vi "REPORT_GEAR_prepare_operations_and_batches_for_csv.vi"(11 "REPORT_GEAR_all_info":T1) -> (2 "report_batches":string[][](array[string]), 3 "report_results":string[][](array[string]))   [LabVIEW 2019]
uses:
  typedef/REPORT_GEAR_all_info.ctl
  typedef/REPORT_GEAR_header_data_display.ctl
  typedef/REPORT_GEAR_statuses.ctl
  _misc/AULocalize/SubVIs/Get Localized Phrase Compact Interface 1D.vi
panel:
  # "GEAR INFO SUMMARY"
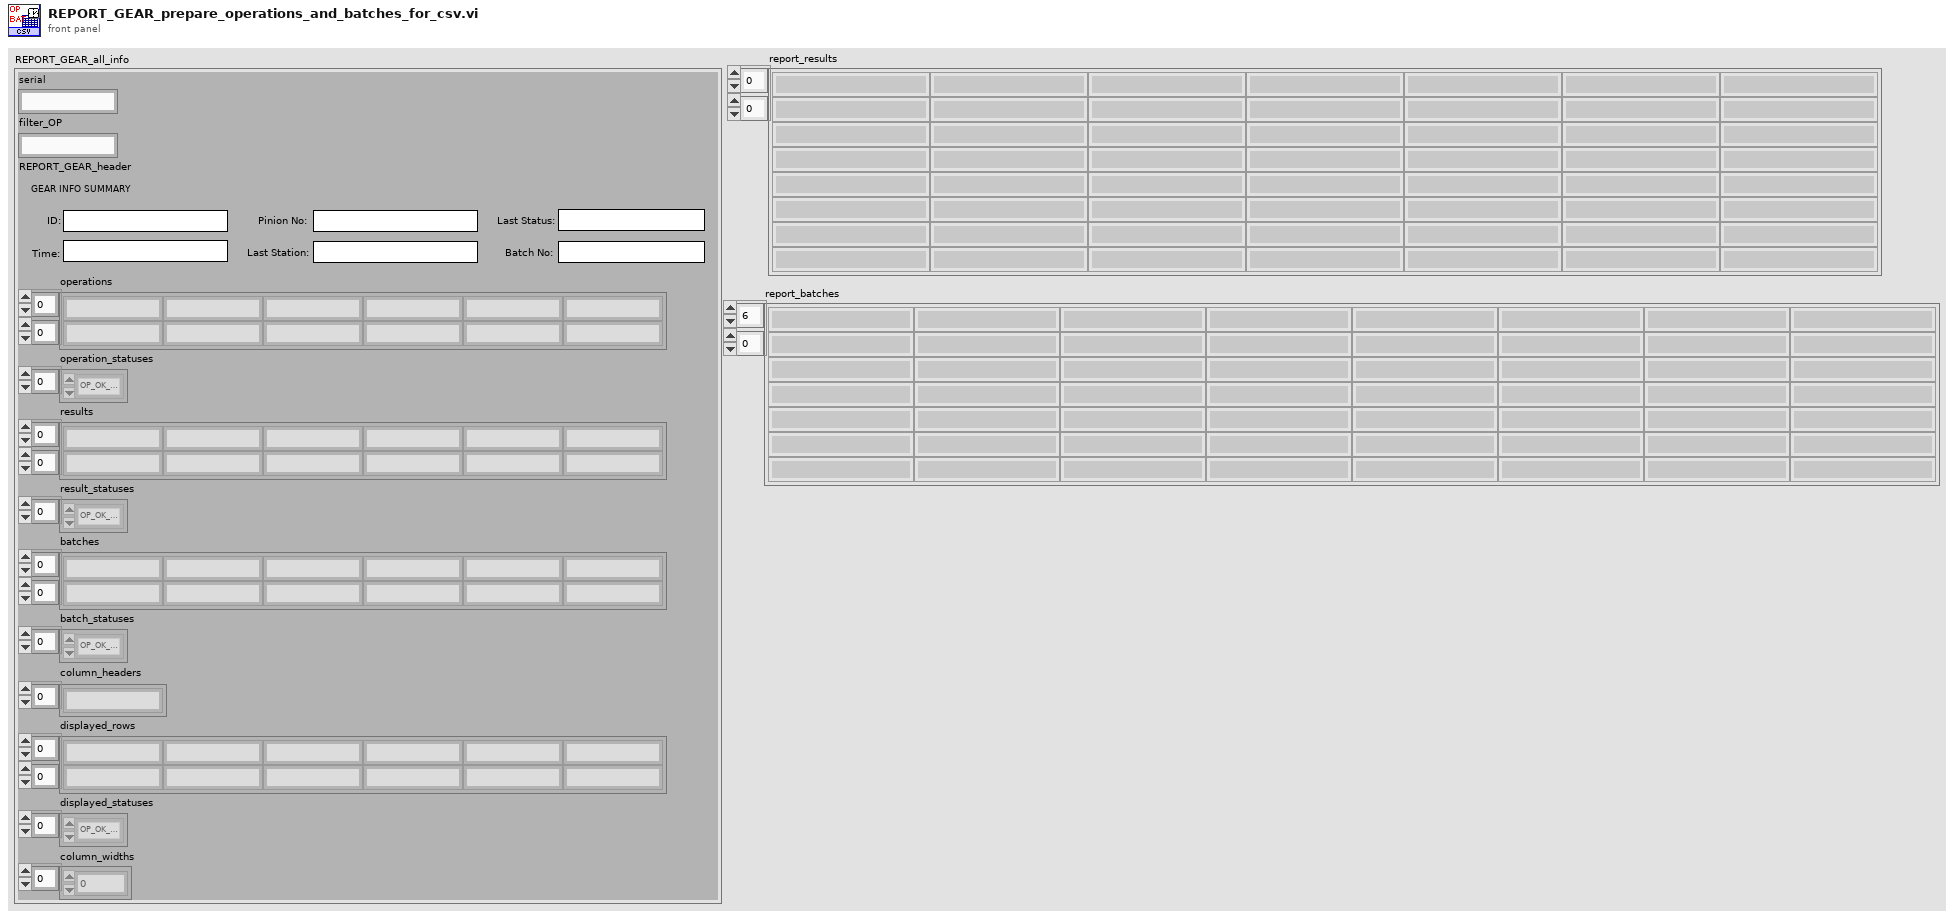
[diagram p1: front panel]
types:
  T1 = typedef "REPORT_GEAR_all_info.ctl" = cluster{"serial":string, "filter_OP":string, "REPORT_GEAR_header":T2, "operations":string[][], "operation_statuses":T3[], "results":string[][], "result_statuses":T3[], "batches":string[][], "batch_statuses":T3[], "column_headers":string[], "displayed_rows":string[][], "displayed_statuses":T3[], "column_widths":i16[]}
  T2 = typedef "REPORT_GEAR_header_data_display.ctl" = cluster{"ID":string, "creation_time":string, "last_station":string, "last_status":string, "pinion_serial":string, "batch_code":string}
  T3 = typedef "REPORT_GEAR_statuses.ctl" = enum16{"OP_OK_hide", "OP_OK_show", "OP_NOK_hide", "OP_NOK_show", "OP_interrupted_hide", "OP_interrupted_show", "OP_in_operation_hide", "OP_in_operation_show", "OP_unexpected_hide", "OP_unexpected_show", "RE_REAL_OK", "RE_REAL_NOK", "RE_STRING", "RE_sub_header", "RE_no_data", "RE_unexpected", "BA_sub_header", "BA_data", "BA_no_data"}
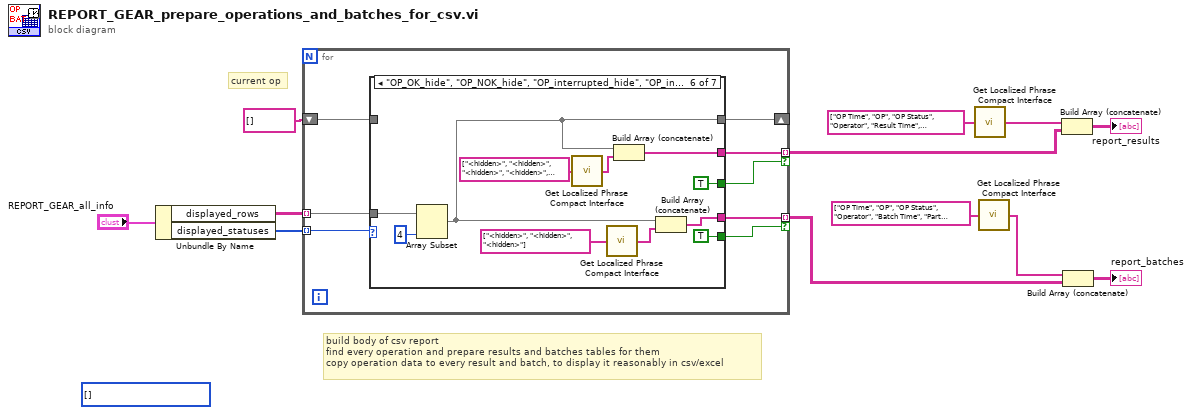
[diagram p0: block diagram]
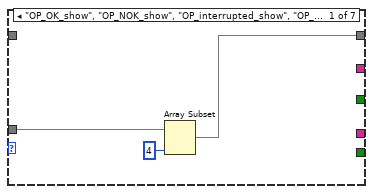
[diagram p2: hidden frame]
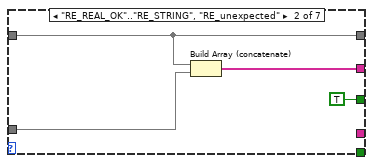
[diagram p3: hidden frame]
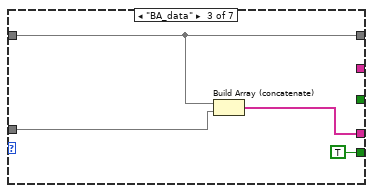
[diagram p4: hidden frame]
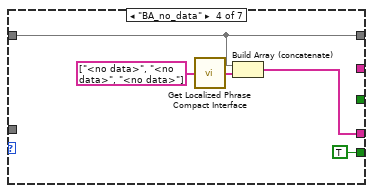
[diagram p5: hidden frame]
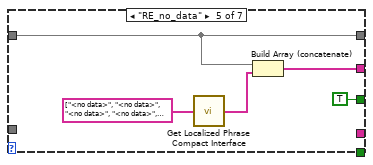
[diagram p6: hidden frame]
diagram:
  (unwired) T3[] [] items=["OP_OK_hide", "OP_OK_show", "OP_NOK_hide", "OP_NOK_show", "OP_interrupted_hide", "OP_interrupted_show", "OP_in_operation_hide", "OP_in_operation_show", "OP_unexpected_hide", "OP_unexpected_show", "RE_REAL_OK", "RE_REAL_NOK", "RE_STRING", "RE_sub_header", "RE_no_data", "RE_unexpected", "BA_sub_header", "BA_data", "BA_no_data"] ("displayed_statuses")
  # "build body of csv report\nfind every operation and prepare results and batches tables for them\ncopy operation data to every result and batch, to display it reasonably in csv/excel"
  # "current op"
  n1 = Unbundle By Name("REPORT_GEAR_all_info") -> ("displayed_rows"=w11:string[][], "displayed_statuses"=w10:T3[])
  n2 = for {
    tunnel: w11 -> [w19] mode=indexing
    tunnel: w10 -> [w20] mode=indexing
    shift-right: [w18] -> _
    shift-left: string[] [] ("displayed_rows") -> [w17]
    tunnel: [w16] -> w4 mode=indexing if=w15
    tunnel: [w14] -> w3 mode=indexing if=w13
    n3 = case shown="\"OP_OK_hide\", \"OP_NOK_hide\", \"OP_interrupted_hide\", \"OP_in_operation_hide\", \"OP_unexpected_hide\"" w20 {
      tunnel: w19 -> [w23 w27 w29 _ _ w43 _]
      tunnel: [w21 w26 w30 w35 w40 w42 w53] -> w18
      tunnel: w17 -> [_ w26 w30 w35 w40 _ w53]
      tunnel: [_ w25 _ _ w38 w51 _] -> w16
      tunnel: [_ TRUE _ _ TRUE TRUE _] -> w15
      tunnel: [_ _ w28 w34 _ w47 _] -> w14
      tunnel: [_ _ TRUE TRUE _ TRUE _] -> w13
      frame "OP_OK_show", "OP_NOK_show", "OP_interrupted_show", "OP_in_operation_show", "OP_unexpected_show" {
        n4 = Array Subset(array=w23, length=4) -> (w21:string[])  [unwired: 1 in]
      }
      frame "RE_REAL_OK".."RE_STRING", "RE_unexpected" {
        n5 = Build Array (concatenate)(w26, w27) -> (w25:string[])
      }
      frame "BA_data" {
        n6 = Build Array (concatenate)(w30, w29) -> (w28:string[])
      }
      frame "BA_no_data" {
        n7 = call-poly "Get Localized Phrase Compact Interface.vi"("Key"=string[] ["<no data>", "<no data>", "<no data>"] ("element")) -> ("Translated Phrase"=w32:string[])
        n8 = Build Array (concatenate)(w35, w32) -> (w34:string[])
      }
      frame "RE_no_data" {
        n9 = call-poly "Get Localized Phrase Compact Interface.vi"("Key"=string[] ["<no data>", "<no data>", "<no data>", "<no data>", "<no data>", "<no data>", "<no data>", "<no data>"] ("element")) -> ("Translated Phrase"=w37:string[])
        n10 = Build Array (concatenate)(w40, w37) -> (w38:string[])
      }
      frame "OP_OK_hide", "OP_NOK_hide", "OP_interrupted_hide", "OP_in_operation_hide", "OP_unexpected_hide" {
        n11 = Array Subset(array=w43, length=4) -> (w42:string[])  [unwired: 1 in]
        n12 = call-poly "Get Localized Phrase Compact Interface.vi"("Key"=string[] ["<hidden>", "<hidden>", "<hidden>", "<hidden>", "<hidden>", "<hidden>", "<hidden>", "<hidden>"] ("element")) -> ("Translated Phrase"=w46:string[])
        n13 = call-poly "Get Localized Phrase Compact Interface.vi"("Key"=string[] ["<hidden>", "<hidden>", "<hidden>"] ("element")) -> ("Translated Phrase"=w45:string[])
        n14 = Build Array (concatenate)(w42, w46) -> (w51:string[])
        n15 = Build Array (concatenate)(w42, w45) -> (w47:string[])
      }
      frame "RE_sub_header", "BA_sub_header" {
      }
    }
  }
  n16 = call-poly "Get Localized Phrase Compact Interface.vi"("Key"=string[] ["OP Time", "OP", "OP Status", "Operator", "Result Time", "Description", "Status", "Type", "Min", "Value", "Max", "Unit"]) -> ("Translated Phrase"=w2:string[])
  n17 = call-poly "Get Localized Phrase Compact Interface.vi"("Key"=string[] ["OP Time", "OP", "OP Status", "Operator", "Batch Time", "Part Number", "Batch Number"]) -> ("Translated Phrase"=w1:string[])
  n18 = Build Array (concatenate)(w2, w4) -> (→"report_results":string[][])
  n19 = Build Array (concatenate)(w1, w3) -> (→"report_batches":string[][])
